vi "StopProgram.vi"(8 "error in (no error)":errorcluster, 9 "task id":i32(ring)=1 items=["TLibrary", "T01", "T02", "T03", "T04", "TAuxiliary"], 11 "controller in":refnum<k24>) -> (0 "error out":errorcluster, 3 "controller out":refnum<k24>)   [LabVIEW 2010]
uses:
  c:/aerotech/controller/5.xx.xxx/ensemble/pc/labview/2010/bin/Aerotech.Ensemble.dll
  bin/Aerotech.Ensemble.dll
  c:/aerotech/controller/5.xx.xxx/ensemble/pc/labview/2010/bin/Aerotech.Ensemble.LabVIEW.dll
  bin/Aerotech.Ensemble.LabVIEW.dll
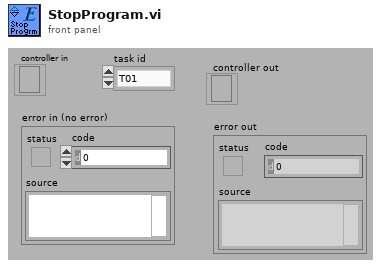
[diagram p1: front panel]
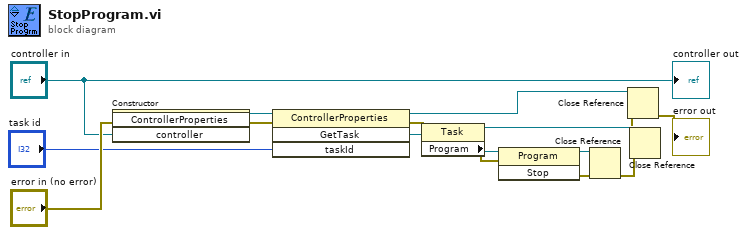
[diagram p0: block diagram]
diagram:
  n1 = constructor class="ControllerProperties"(error in="error in (no error)", "controller"="controller in") -> (reference out=w13:refnum<k24>, error out=w12:errorcluster)  [unwired: 2 in, 2 out]
  n2 = invoke class="ControllerProperties" method="GetTask"(reference=w13, error in=w12, "taskId"="task id") -> (reference out=w11:refnum<k24>, error out=w8:errorcluster, "GetTask"=w9:refnum<k24>)  [unwired: 1 in, 1 out]
  n3 = property class="Task"(reference=w9, error in=w8) -> (reference out=w3:refnum<k24>, error out=w2:errorcluster, "Program"=w6:refnum<k24>)
  n4 = invoke class="Program" method="Stop"(reference=w6, error in=w2) -> (reference out=w5:refnum<k24>, error out=w4:errorcluster)  [unwired: 1 in, 1 out]
  n5 = Close Reference(reference=w5, error in (no error)=w4) -> (error out=w7:errorcluster)
  n6 = Close Reference(reference=w3, error in (no error)=w7) -> (error out=w1:errorcluster)
  n7 = Close Reference(reference=w11, error in (no error)=w1) -> (error out=→"error out":errorcluster)
  "controller out" <- "controller in"
